vi "SetListWindowVisible.vi"(0 "Display State In":T1, 5 "Visible":bool, 9 "Container State":T2, 11 "error in (no error)":errorcluster) -> (4 "Display State Out":T1, 15 "error out":errorcluster)   [LabVIEW 2017, in "XListGraph.lvlib" / "XListGraph.xctl"]
uses:
  XListGraph.xctl
  <vilib>/_xctls/Container State.ctl
  Ability/State.ctl
  Support/def-XListGraphOper.ctl
  <vilib>/_xctls/XControlSupport.lvlib
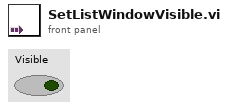
[diagram p1: front panel]
types:
  T1 = typedef "XListGraph.lvlib/XListGraph.xctl/State.ctl" = cluster{"ListWindowSpliterPos":i32, "ListWindowSpliterLocked":bool, "axes":cluster{"X":cluster{"Label":string, "Unit":string}, "Y":cluster{"Label":string, "Unit":string}}, "Next State":string, "User Event":refnum<user-event>, "Plot Names":string[], "Visible Plot Names":string[], "Selected Plot Names":string[]}
  T2 = typedef "XControlSupport.lvlib/Container State.ctl" = cluster{"Indicator?":bool, "Run Mode?":bool, " Refnum":refnum<vi>}
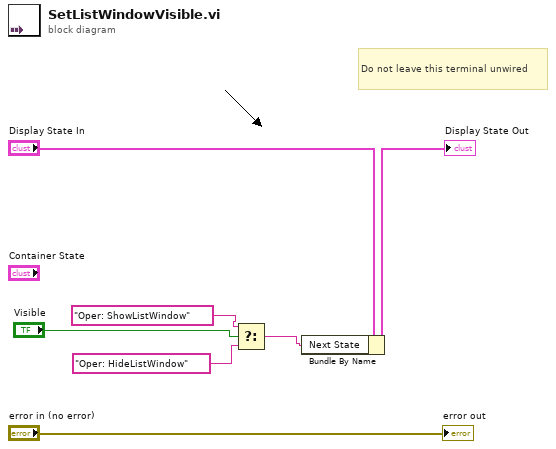
[diagram p0: block diagram]
diagram:
  # "Do not leave this terminal unwired"
  n1 = Select(t="Oper: ShowListWindow", s="Visible", f="Oper: HideListWindow") -> (s? t:f=w1:string)
  n2 = Bundle By Name(cluster="Display State In", "Next State"=w1) -> (→"Display State Out":T1)
  "error out" <- "error in (no error)"
